vi "data_generation.vi"(0 "X Size":i32=8, 1 "slope":i16=10, 3 "scan range (um)":dbl=5.0, 4 "AmplitudeX":dbl=1.0, 5 "AmplitudeY":dbl=1.0, 6 "dwell time":i16=10, 7 "come back":i32, 8 "calibration":dbl=5.0, 9 "multicolor":dbl=5.0, 10 "zero point":dbl, 12 "first":dbl=0.5, 13 "Y size":i32=8, 15 "AmplitudeC":dbl=1.0, 17 "step size (um)":dbl=0.05, 18 "Samples per spot":i32=4, 19 "zero point 2":dbl) -> (2 "Output Graph":waveform(dbl)[](graph), 11 "DO":dbl[](array[numeric])=[0.0, 0.0, 0.0, 0.0, 0.0, 0.0, 0.0, 0.0, 1.0, 1.0, 1.0, 1.0, 1.0, 1.0, 1.0, 1.0, 2.0, 2.0, 2.0, 2.0, 2.0, 2.0, 2.0, 2.0, 3.0, 3.0, 3.0, 3.0, 3.0, 3.0, 3.0, 3.0, 4.0, 4.0, 4.0, 4.0, 4.0, 4.0, 4.0, 4.0, 5.0, 5.0, 5.0, 5.0, 5.0, 5.0, 5.0, 5.0, 6.0, 6.0, 6.0, 6.0, 6.0, 6.0, 6.0, 6.0, 7.0, 7.0, 7.0, 7.0, 7.0, 7.0, 7.0, 7.0, 7.0, 7.0, 7.0, 7.0, 7.0, 7.0, 7.0, 7.0, 6.0, 6.0, 6.0, 6.0, 6.0, 6.0, 6.0, 6.0, 5.0, 5.0, 5.0, 5.0, 5.0, 5.0, 5.0, 5.0, 4.0, 4.0, 4.0, 4.0, 4.0, 4.0, 4.0, 4.0, 3.0, 3.0, 3.0, 3.0, 3.0, 3.0, 3.0, 3.0, 2.0, 2.0, 2.0, 2.0, 2.0, 2.0, 2.0, 2.0, 1.0, 1.0, 1.0, 1.0, 1.0, 1.0, 1.0, 1.0, 0.0, 0.0, 0.0, 0.0, 0.0, 0.0, 0.0, 0.0], 14 "XY Scan":waveform(dbl)[](array[waveform])=[{"t0"=timestamp(3264022747.299 s since 1904-01-01), "dt"=0.015625, "Y"=[-1.0, -0.7142857142857143, -0.4285714285714286, -0.1428571428571429, 0.1428571428571428, 0.4285714285714286, 0.7142857142857142, 1.0, 1.0, 0.7142857142857142, 0.4285714285714286, 0.1428571428571428, -0.1428571428571429, -0.4285714285714286, -0.7142857142857143, -1.0, -1.0, -0.7142857142857143, -0.4285714285714286, -0.1428571428571429, 0.1428571428571428, 0.4285714285714286, 0.7142857142857142, 1.0, 1.0, 0.7142857142857142, 0.4285714285714286, 0.1428571428571428, -0.1428571428571429, -0.4285714285714286, -0.7142857142857143, -1.0, -1.0, -0.7142857142857143, -0.4285714285714286, -0.1428571428571429, 0.1428571428571428, 0.4285714285714286, 0.7142857142857142, 1.0, 1.0, 0.7142857142857142, 0.4285714285714286, 0.1428571428571428, -0.1428571428571429, -0.4285714285714286, -0.7142857142857143, -1.0, -1.0, -0.7142857142857143, -0.4285714285714286, -0.1428571428571429, 0.1428571428571428, 0.4285714285714286, 0.7142857142857142, 1.0, 1.0, 0.7142857142857142, 0.4285714285714286, 0.1428571428571428, -0.1428571428571429, -0.4285714285714286, -0.7142857142857143, -1.0, -1.0, -0.7142857142857143, -0.4285714285714286, -0.1428571428571429, 0.1428571428571428, 0.4285714285714286, 0.7142857142857142, 1.0, 1.0, 0.7142857142857142, 0.4285714285714286, 0.1428571428571428, -0.1428571428571429, -0.4285714285714286, -0.7142857142857143, -1.0, -1.0, -0.7142857142857143, -0.4285714285714286, -0.1428571428571429, 0.1428571428571428, 0.4285714285714286, 0.7142857142857142, 1.0, 1.0, 0.7142857142857142, 0.4285714285714286, 0.1428571428571428, -0.1428571428571429, -0.4285714285714286, -0.7142857142857143, -1.0, -1.0, -0.7142857142857143, -0.4285714285714286, -0.1428571428571429, 0.1428571428571428, 0.4285714285714286, 0.7142857142857142, 1.0, 1.0, 0.7142857142857142, 0.4285714285714286, 0.1428571428571428, -0.1428571428571429, -0.4285714285714286, -0.7142857142857143, -1.0, -1.0, -0.7142857142857143, -0.4285714285714286, -0.1428571428571429, 0.1428571428571428, 0.4285714285714286, 0.7142857142857142, 1.0, 1.0, 0.7142857142857142, 0.4285714285714286, 0.1428571428571428, -0.1428571428571429, -0.4285714285714286, -0.7142857142857143, -1.0]}, {"t0"=timestamp(3264022747.299 s since 1904-01-01), "dt"=0.015625, "Y"=[-1.0, -1.0, -1.0, -1.0, -1.0, -1.0, -1.0, -1.0, -0.7142857142857143, -0.7142857142857143, -0.7142857142857143, -0.7142857142857143, -0.7142857142857143, -0.7142857142857143, -0.7142857142857143, -0.7142857142857143, -0.4285714285714286, -0.4285714285714286, -0.4285714285714286, -0.4285714285714286, -0.4285714285714286, -0.4285714285714286, -0.4285714285714286, -0.4285714285714286, -0.1428571428571429, -0.1428571428571429, -0.1428571428571429, -0.1428571428571429, -0.1428571428571429, -0.1428571428571429, -0.1428571428571429, -0.1428571428571429, 0.1428571428571428, 0.1428571428571428, 0.1428571428571428, 0.1428571428571428, 0.1428571428571428, 0.1428571428571428, 0.1428571428571428, 0.1428571428571428, 0.4285714285714286, 0.4285714285714286, 0.4285714285714286, 0.4285714285714286, 0.4285714285714286, 0.4285714285714286, 0.4285714285714286, 0.4285714285714286, 0.7142857142857142, 0.7142857142857142, 0.7142857142857142, 0.7142857142857142, 0.7142857142857142, 0.7142857142857142, 0.7142857142857142, 0.7142857142857142, 1.0, 1.0, 1.0, 1.0, 1.0, 1.0, 1.0, 1.0, 1.0, 1.0, 1.0, 1.0, 1.0, 1.0, 1.0, 1.0, 0.7142857142857142, 0.7142857142857142, 0.7142857142857142, 0.7142857142857142, 0.7142857142857142, 0.7142857142857142, 0.7142857142857142, 0.7142857142857142, 0.4285714285714286, 0.4285714285714286, 0.4285714285714286, 0.4285714285714286, 0.4285714285714286, 0.4285714285714286, 0.4285714285714286, 0.4285714285714286, 0.1428571428571428, 0.1428571428571428, 0.1428571428571428, 0.1428571428571428, 0.1428571428571428, 0.1428571428571428, 0.1428571428571428, 0.1428571428571428, -0.1428571428571429, -0.1428571428571429, -0.1428571428571429, -0.1428571428571429, -0.1428571428571429, -0.1428571428571429, -0.1428571428571429, -0.1428571428571429, -0.4285714285714286, -0.4285714285714286, -0.4285714285714286, -0.4285714285714286, -0.4285714285714286, -0.4285714285714286, -0.4285714285714286, -0.4285714285714286, -0.7142857142857143, -0.7142857142857143, -0.7142857142857143, -0.7142857142857143, -0.7142857142857143, -0.7142857142857143, -0.7142857142857143, -0.7142857142857143, -1.0, -1.0, -1.0, -1.0, -1.0, -1.0, -1.0, -1.0]}])   [LabVIEW 2017]
uses:
  <vilib>/Analysis/3filter.llb/Zero Phase Filter (DBL).vi
  <vilib>/Analysis/NI_AALBase.lvlib
panel:
  out "AO Data":dbl[][](array[numeric])
  out "nanoZ output":dbl[](array[numeric])=[-1.0, -1.0, -1.0, -1.0, -1.0, -1.0, -1.0, -1.0, -0.7142857142857143, -0.7142857142857143, -0.7142857142857143, -0.7142857142857143, -0.7142857142857143, -0.7142857142857143, -0.7142857142857143, -0.7142857142857143, -0.4285714285714286, -0.4285714285714286, -0.4285714285714286, -0.4285714285714286, -0.4285714285714286, -0.4285714285714286, -0.4285714285714286, -0.4285714285714286, -0.1428571428571429, -0.1428571428571429, -0.1428571428571429, -0.1428571428571429, -0.1428571428571429, -0.1428571428571429, -0.1428571428571429, -0.1428571428571429, 0.1428571428571428, 0.1428571428571428, 0.1428571428571428, 0.1428571428571428, 0.1428571428571428, 0.1428571428571428, 0.1428571428571428, 0.1428571428571428, 0.4285714285714286, 0.4285714285714286, 0.4285714285714286, 0.4285714285714286, 0.4285714285714286, 0.4285714285714286, 0.4285714285714286, 0.4285714285714286, 0.7142857142857142, 0.7142857142857142, 0.7142857142857142, 0.7142857142857142, 0.7142857142857142, 0.7142857142857142, 0.7142857142857142, 0.7142857142857142, 1.0, 1.0, 1.0, 1.0, 1.0, 1.0, 1.0, 1.0, 1.0, 1.0, 1.0, 1.0, 1.0, 1.0, 1.0, 1.0, 0.7142857142857142, 0.7142857142857142, 0.7142857142857142, 0.7142857142857142, 0.7142857142857142, 0.7142857142857142, 0.7142857142857142, 0.7142857142857142, 0.4285714285714286, 0.4285714285714286, 0.4285714285714286, 0.4285714285714286, 0.4285714285714286, 0.4285714285714286, 0.4285714285714286, 0.4285714285714286, 0.1428571428571428, 0.1428571428571428, 0.1428571428571428, 0.1428571428571428, 0.1428571428571428, 0.1428571428571428, 0.1428571428571428, 0.1428571428571428, -0.1428571428571429, -0.1428571428571429, -0.1428571428571429, -0.1428571428571429, -0.1428571428571429, -0.1428571428571429, -0.1428571428571429, -0.1428571428571429, -0.4285714285714286, -0.4285714285714286, -0.4285714285714286, -0.4285714285714286, -0.4285714285714286, -0.4285714285714286, -0.4285714285714286, -0.4285714285714286, -0.7142857142857143, -0.7142857142857143, -0.7142857142857143, -0.7142857142857143, -0.7142857142857143, -0.7142857142857143, -0.7142857142857143, -0.7142857142857143, -1.0, -1.0, -1.0, -1.0, -1.0, -1.0, -1.0, -1.0]
  out "nanoZ":dbl[](array[numeric])=[0.0, 1.0, 2.0, 3.0, 4.0, 5.0, 6.0, 7.0, 7.0, 6.0, 5.0, 4.0, 3.0, 2.0, 1.0, 0.0, 0.0, 1.0, 2.0, 3.0, 4.0, 5.0, 6.0, 7.0, 7.0, 6.0, 5.0, 4.0, 3.0, 2.0, 1.0, 0.0, 0.0, 1.0, 2.0, 3.0, 4.0, 5.0, 6.0, 7.0, 7.0, 6.0, 5.0, 4.0, 3.0, 2.0, 1.0, 0.0, 0.0, 1.0, 2.0, 3.0, 4.0, 5.0, 6.0, 7.0, 7.0, 6.0, 5.0, 4.0, 3.0, 2.0, 1.0, 0.0, 0.0, 1.0, 2.0, 3.0, 4.0, 5.0, 6.0, 7.0, 7.0, 6.0, 5.0, 4.0, 3.0, 2.0, 1.0, 0.0, 0.0, 1.0, 2.0, 3.0, 4.0, 5.0, 6.0, 7.0, 7.0, 6.0, 5.0, 4.0, 3.0, 2.0, 1.0, 0.0, 0.0, 1.0, 2.0, 3.0, 4.0, 5.0, 6.0, 7.0, 7.0, 6.0, 5.0, 4.0, 3.0, 2.0, 1.0, 0.0, 0.0, 1.0, 2.0, 3.0, 4.0, 5.0, 6.0, 7.0, 7.0, 6.0, 5.0, 4.0, 3.0, 2.0, 1.0, 0.0]
  out "Trigger output":dbl[](array[numeric])=[-1.0, -1.0, -1.0, -1.0, -1.0, -1.0, -1.0, -1.0, -0.7142857142857143, -0.7142857142857143, -0.7142857142857143, -0.7142857142857143, -0.7142857142857143, -0.7142857142857143, -0.7142857142857143, -0.7142857142857143, -0.4285714285714286, -0.4285714285714286, -0.4285714285714286, -0.4285714285714286, -0.4285714285714286, -0.4285714285714286, -0.4285714285714286, -0.4285714285714286, -0.1428571428571429, -0.1428571428571429, -0.1428571428571429, -0.1428571428571429, -0.1428571428571429, -0.1428571428571429, -0.1428571428571429, -0.1428571428571429, 0.1428571428571428, 0.1428571428571428, 0.1428571428571428, 0.1428571428571428, 0.1428571428571428, 0.1428571428571428, 0.1428571428571428, 0.1428571428571428, 0.4285714285714286, 0.4285714285714286, 0.4285714285714286, 0.4285714285714286, 0.4285714285714286, 0.4285714285714286, 0.4285714285714286, 0.4285714285714286, 0.7142857142857142, 0.7142857142857142, 0.7142857142857142, 0.7142857142857142, 0.7142857142857142, 0.7142857142857142, 0.7142857142857142, 0.7142857142857142, 1.0, 1.0, 1.0, 1.0, 1.0, 1.0, 1.0, 1.0, 1.0, 1.0, 1.0, 1.0, 1.0, 1.0, 1.0, 1.0, 0.7142857142857142, 0.7142857142857142, 0.7142857142857142, 0.7142857142857142, 0.7142857142857142, 0.7142857142857142, 0.7142857142857142, 0.7142857142857142, 0.4285714285714286, 0.4285714285714286, 0.4285714285714286, 0.4285714285714286, 0.4285714285714286, 0.4285714285714286, 0.4285714285714286, 0.4285714285714286, 0.1428571428571428, 0.1428571428571428, 0.1428571428571428, 0.1428571428571428, 0.1428571428571428, 0.1428571428571428, 0.1428571428571428, 0.1428571428571428, -0.1428571428571429, -0.1428571428571429, -0.1428571428571429, -0.1428571428571429, -0.1428571428571429, -0.1428571428571429, -0.1428571428571429, -0.1428571428571429, -0.4285714285714286, -0.4285714285714286, -0.4285714285714286, -0.4285714285714286, -0.4285714285714286, -0.4285714285714286, -0.4285714285714286, -0.4285714285714286, -0.7142857142857143, -0.7142857142857143, -0.7142857142857143, -0.7142857142857143, -0.7142857142857143, -0.7142857142857143, -0.7142857142857143, -0.7142857142857143, -1.0, -1.0, -1.0, -1.0, -1.0, -1.0, -1.0, -1.0]
  out "Trigger":dbl[](array[numeric])=[0.0, 0.0, 0.0, 0.0, 0.0, 0.0, 0.0, 0.0, 1.0, 1.0, 1.0, 1.0, 1.0, 1.0, 1.0, 1.0, 2.0, 2.0, 2.0, 2.0, 2.0, 2.0, 2.0, 2.0, 3.0, 3.0, 3.0, 3.0, 3.0, 3.0, 3.0, 3.0, 4.0, 4.0, 4.0, 4.0, 4.0, 4.0, 4.0, 4.0, 5.0, 5.0, 5.0, 5.0, 5.0, 5.0, 5.0, 5.0, 6.0, 6.0, 6.0, 6.0, 6.0, 6.0, 6.0, 6.0, 7.0, 7.0, 7.0, 7.0, 7.0, 7.0, 7.0, 7.0, 7.0, 7.0, 7.0, 7.0, 7.0, 7.0, 7.0, 7.0, 6.0, 6.0, 6.0, 6.0, 6.0, 6.0, 6.0, 6.0, 5.0, 5.0, 5.0, 5.0, 5.0, 5.0, 5.0, 5.0, 4.0, 4.0, 4.0, 4.0, 4.0, 4.0, 4.0, 4.0, 3.0, 3.0, 3.0, 3.0, 3.0, 3.0, 3.0, 3.0, 2.0, 2.0, 2.0, 2.0, 2.0, 2.0, 2.0, 2.0, 1.0, 1.0, 1.0, 1.0, 1.0, 1.0, 1.0, 1.0, 0.0, 0.0, 0.0, 0.0, 0.0, 0.0, 0.0, 0.0]
  in  "dt":dbl=1e-05
  out "time":dbl=3264022747.299 format="%<%I:%M:%S %p\n%m/%d/%Y>T"
  out "Y output Array":dbl[](array[numeric])=[-1.0, -1.0, -1.0, -1.0, -1.0, -1.0, -1.0, -1.0, -0.7142857142857143, -0.7142857142857143, -0.7142857142857143, -0.7142857142857143, -0.7142857142857143, -0.7142857142857143, -0.7142857142857143, -0.7142857142857143, -0.4285714285714286, -0.4285714285714286, -0.4285714285714286, -0.4285714285714286, -0.4285714285714286, -0.4285714285714286, -0.4285714285714286, -0.4285714285714286, -0.1428571428571429, -0.1428571428571429, -0.1428571428571429, -0.1428571428571429, -0.1428571428571429, -0.1428571428571429, -0.1428571428571429, -0.1428571428571429, 0.1428571428571428, 0.1428571428571428, 0.1428571428571428, 0.1428571428571428, 0.1428571428571428, 0.1428571428571428, 0.1428571428571428, 0.1428571428571428, 0.4285714285714286, 0.4285714285714286, 0.4285714285714286, 0.4285714285714286, 0.4285714285714286, 0.4285714285714286, 0.4285714285714286, 0.4285714285714286, 0.7142857142857142, 0.7142857142857142, 0.7142857142857142, 0.7142857142857142, 0.7142857142857142, 0.7142857142857142, 0.7142857142857142, 0.7142857142857142, 1.0, 1.0, 1.0, 1.0, 1.0, 1.0, 1.0, 1.0, 1.0, 1.0, 1.0, 1.0, 1.0, 1.0, 1.0, 1.0, 0.7142857142857142, 0.7142857142857142, 0.7142857142857142, 0.7142857142857142, 0.7142857142857142, 0.7142857142857142, 0.7142857142857142, 0.7142857142857142, 0.4285714285714286, 0.4285714285714286, 0.4285714285714286, 0.4285714285714286, 0.4285714285714286, 0.4285714285714286, 0.4285714285714286, 0.4285714285714286, 0.1428571428571428, 0.1428571428571428, 0.1428571428571428, 0.1428571428571428, 0.1428571428571428, 0.1428571428571428, 0.1428571428571428, 0.1428571428571428, -0.1428571428571429, -0.1428571428571429, -0.1428571428571429, -0.1428571428571429, -0.1428571428571429, -0.1428571428571429, -0.1428571428571429, -0.1428571428571429, -0.4285714285714286, -0.4285714285714286, -0.4285714285714286, -0.4285714285714286, -0.4285714285714286, -0.4285714285714286, -0.4285714285714286, -0.4285714285714286, -0.7142857142857143, -0.7142857142857143, -0.7142857142857143, -0.7142857142857143, -0.7142857142857143, -0.7142857142857143, -0.7142857142857143, -0.7142857142857143, -1.0, -1.0, -1.0, -1.0, -1.0, -1.0, -1.0, -1.0]
  out "X output Array":dbl[](array[numeric])=[-1.0, -0.7142857142857143, -0.4285714285714286, -0.1428571428571429, 0.1428571428571428, 0.4285714285714286, 0.7142857142857142, 1.0, 1.0, 0.7142857142857142, 0.4285714285714286, 0.1428571428571428, -0.1428571428571429, -0.4285714285714286, -0.7142857142857143, -1.0, -1.0, -0.7142857142857143, -0.4285714285714286, -0.1428571428571429, 0.1428571428571428, 0.4285714285714286, 0.7142857142857142, 1.0, 1.0, 0.7142857142857142, 0.4285714285714286, 0.1428571428571428, -0.1428571428571429, -0.4285714285714286, -0.7142857142857143, -1.0, -1.0, -0.7142857142857143, -0.4285714285714286, -0.1428571428571429, 0.1428571428571428, 0.4285714285714286, 0.7142857142857142, 1.0, 1.0, 0.7142857142857142, 0.4285714285714286, 0.1428571428571428, -0.1428571428571429, -0.4285714285714286, -0.7142857142857143, -1.0, -1.0, -0.7142857142857143, -0.4285714285714286, -0.1428571428571429, 0.1428571428571428, 0.4285714285714286, 0.7142857142857142, 1.0, 1.0, 0.7142857142857142, 0.4285714285714286, 0.1428571428571428, -0.1428571428571429, -0.4285714285714286, -0.7142857142857143, -1.0, -1.0, -0.7142857142857143, -0.4285714285714286, -0.1428571428571429, 0.1428571428571428, 0.4285714285714286, 0.7142857142857142, 1.0, 1.0, 0.7142857142857142, 0.4285714285714286, 0.1428571428571428, -0.1428571428571429, -0.4285714285714286, -0.7142857142857143, -1.0, -1.0, -0.7142857142857143, -0.4285714285714286, -0.1428571428571429, 0.1428571428571428, 0.4285714285714286, 0.7142857142857142, 1.0, 1.0, 0.7142857142857142, 0.4285714285714286, 0.1428571428571428, -0.1428571428571429, -0.4285714285714286, -0.7142857142857143, -1.0, -1.0, -0.7142857142857143, -0.4285714285714286, -0.1428571428571429, 0.1428571428571428, 0.4285714285714286, 0.7142857142857142, 1.0, 1.0, 0.7142857142857142, 0.4285714285714286, 0.1428571428571428, -0.1428571428571429, -0.4285714285714286, -0.7142857142857143, -1.0, -1.0, -0.7142857142857143, -0.4285714285714286, -0.1428571428571429, 0.1428571428571428, 0.4285714285714286, 0.7142857142857142, 1.0, 1.0, 0.7142857142857142, 0.4285714285714286, 0.1428571428571428, -0.1428571428571429, -0.4285714285714286, -0.7142857142857143, -1.0]
  out "Y index Array":dbl[](array[numeric])=[0.0, 0.0, 0.0, 0.0, 0.0, 0.0, 0.0, 0.0, 1.0, 1.0, 1.0, 1.0, 1.0, 1.0, 1.0, 1.0, 2.0, 2.0, 2.0, 2.0, 2.0, 2.0, 2.0, 2.0, 3.0, 3.0, 3.0, 3.0, 3.0, 3.0, 3.0, 3.0, 4.0, 4.0, 4.0, 4.0, 4.0, 4.0, 4.0, 4.0, 5.0, 5.0, 5.0, 5.0, 5.0, 5.0, 5.0, 5.0, 6.0, 6.0, 6.0, 6.0, 6.0, 6.0, 6.0, 6.0, 7.0, 7.0, 7.0, 7.0, 7.0, 7.0, 7.0, 7.0, 7.0, 7.0, 7.0, 7.0, 7.0, 7.0, 7.0, 7.0, 6.0, 6.0, 6.0, 6.0, 6.0, 6.0, 6.0, 6.0, 5.0, 5.0, 5.0, 5.0, 5.0, 5.0, 5.0, 5.0, 4.0, 4.0, 4.0, 4.0, 4.0, 4.0, 4.0, 4.0, 3.0, 3.0, 3.0, 3.0, 3.0, 3.0, 3.0, 3.0, 2.0, 2.0, 2.0, 2.0, 2.0, 2.0, 2.0, 2.0, 1.0, 1.0, 1.0, 1.0, 1.0, 1.0, 1.0, 1.0, 0.0, 0.0, 0.0, 0.0, 0.0, 0.0, 0.0, 0.0]
  out "X index Array":dbl[](array[numeric])=[0.0, 1.0, 2.0, 3.0, 4.0, 5.0, 6.0, 7.0, 7.0, 6.0, 5.0, 4.0, 3.0, 2.0, 1.0, 0.0, 0.0, 1.0, 2.0, 3.0, 4.0, 5.0, 6.0, 7.0, 7.0, 6.0, 5.0, 4.0, 3.0, 2.0, 1.0, 0.0, 0.0, 1.0, 2.0, 3.0, 4.0, 5.0, 6.0, 7.0, 7.0, 6.0, 5.0, 4.0, 3.0, 2.0, 1.0, 0.0, 0.0, 1.0, 2.0, 3.0, 4.0, 5.0, 6.0, 7.0, 7.0, 6.0, 5.0, 4.0, 3.0, 2.0, 1.0, 0.0, 0.0, 1.0, 2.0, 3.0, 4.0, 5.0, 6.0, 7.0, 7.0, 6.0, 5.0, 4.0, 3.0, 2.0, 1.0, 0.0, 0.0, 1.0, 2.0, 3.0, 4.0, 5.0, 6.0, 7.0, 7.0, 6.0, 5.0, 4.0, 3.0, 2.0, 1.0, 0.0, 0.0, 1.0, 2.0, 3.0, 4.0, 5.0, 6.0, 7.0, 7.0, 6.0, 5.0, 4.0, 3.0, 2.0, 1.0, 0.0, 0.0, 1.0, 2.0, 3.0, 4.0, 5.0, 6.0, 7.0, 7.0, 6.0, 5.0, 4.0, 3.0, 2.0, 1.0, 0.0]
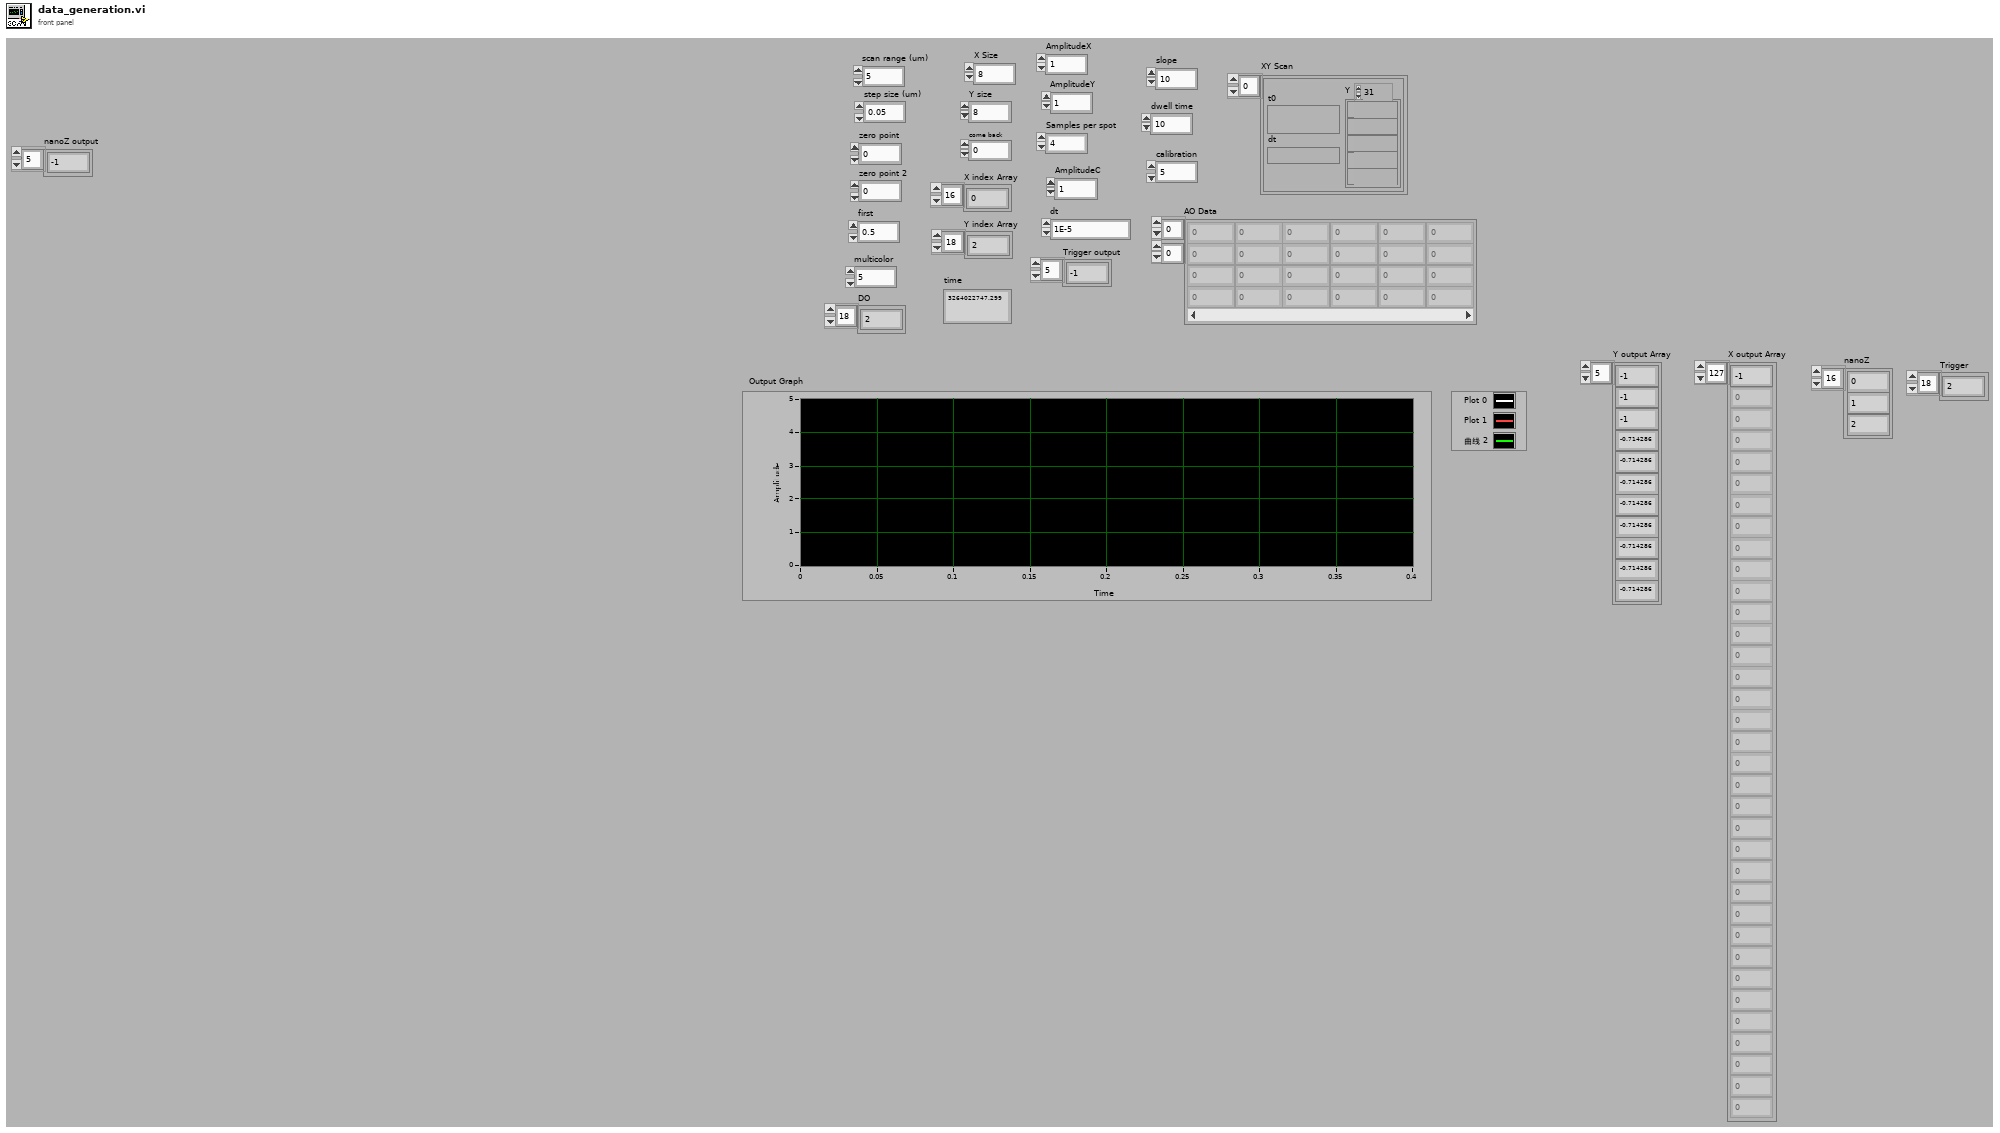
[diagram p1: front panel]
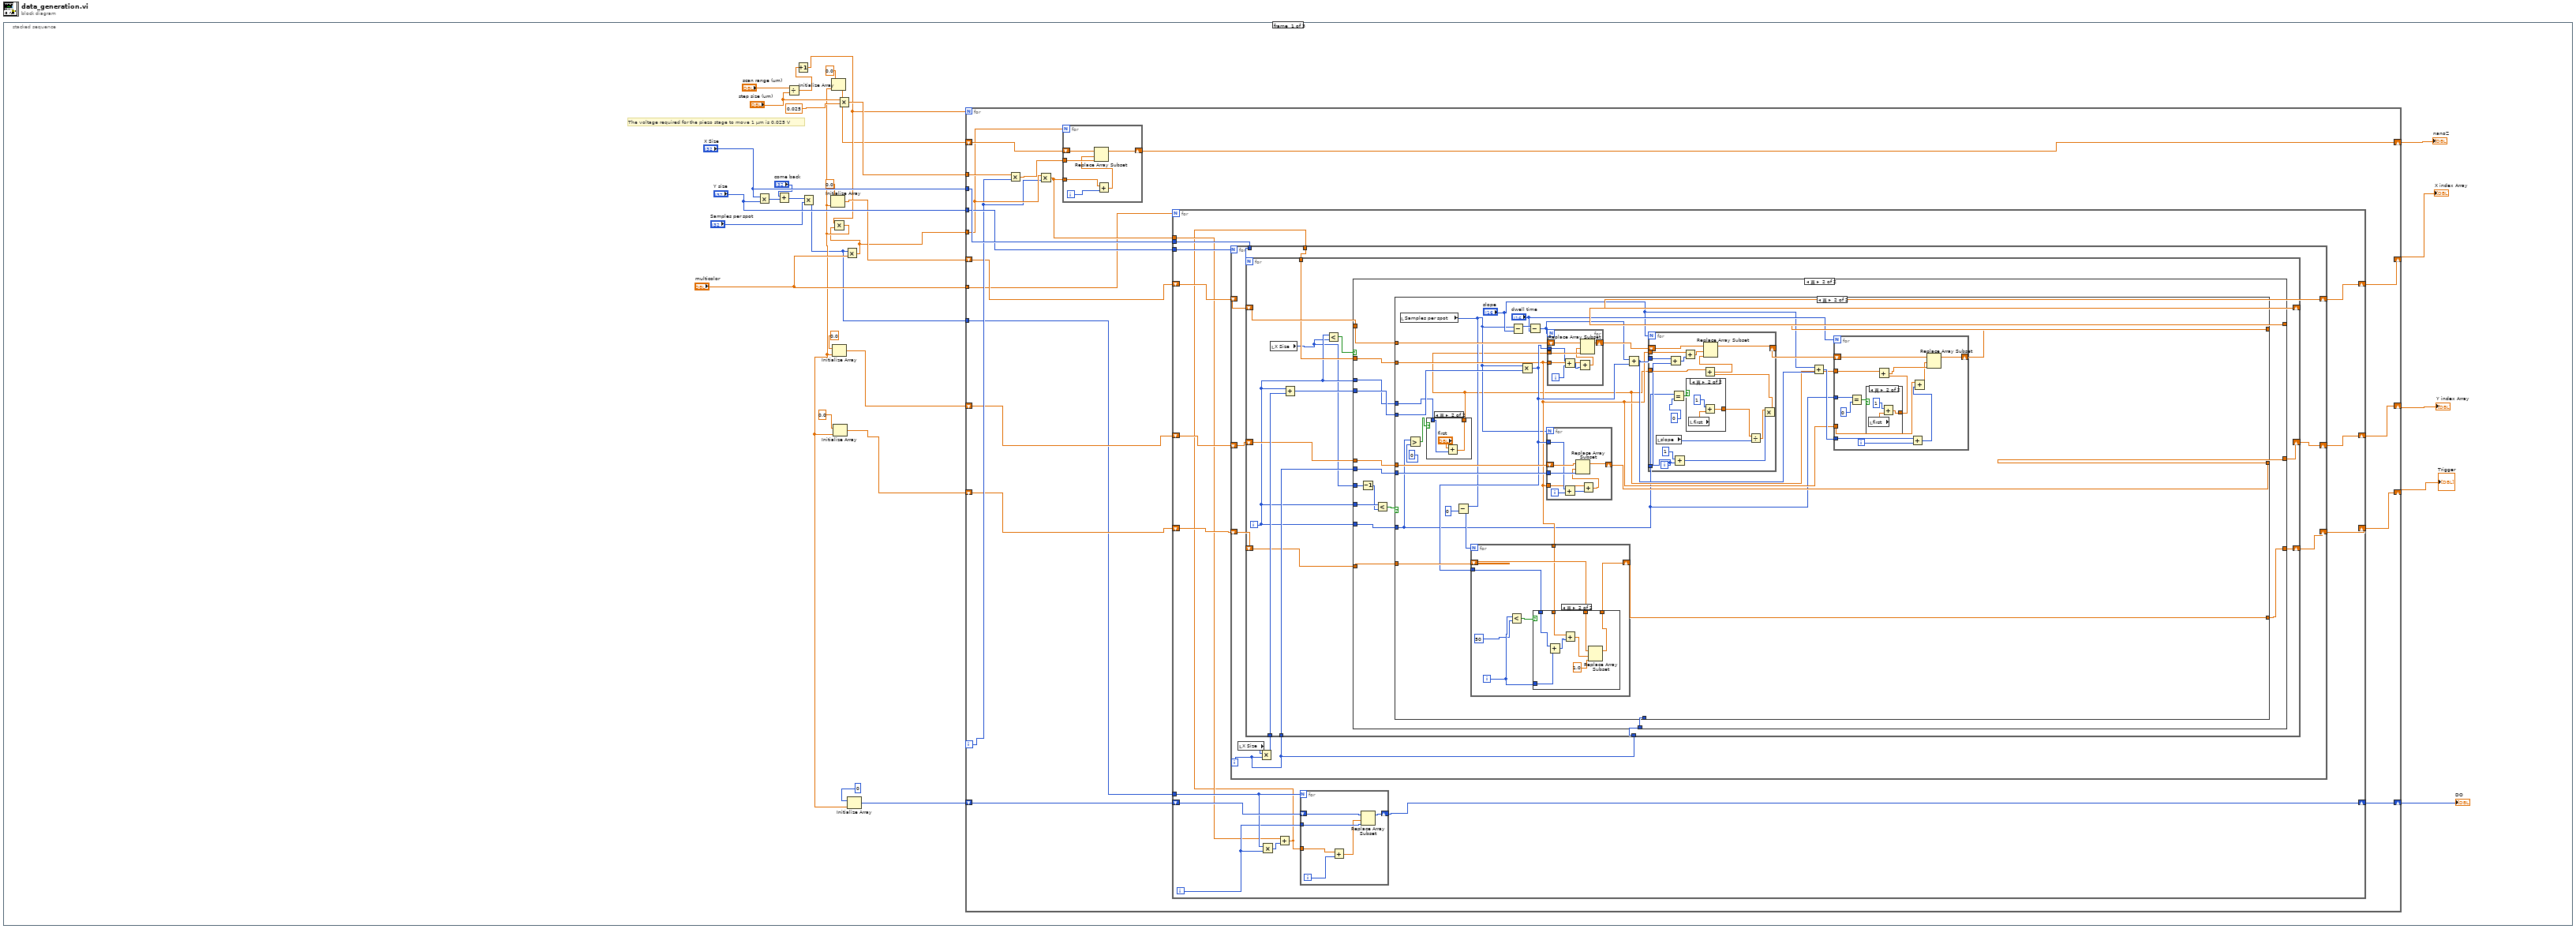
[diagram p0: block diagram]
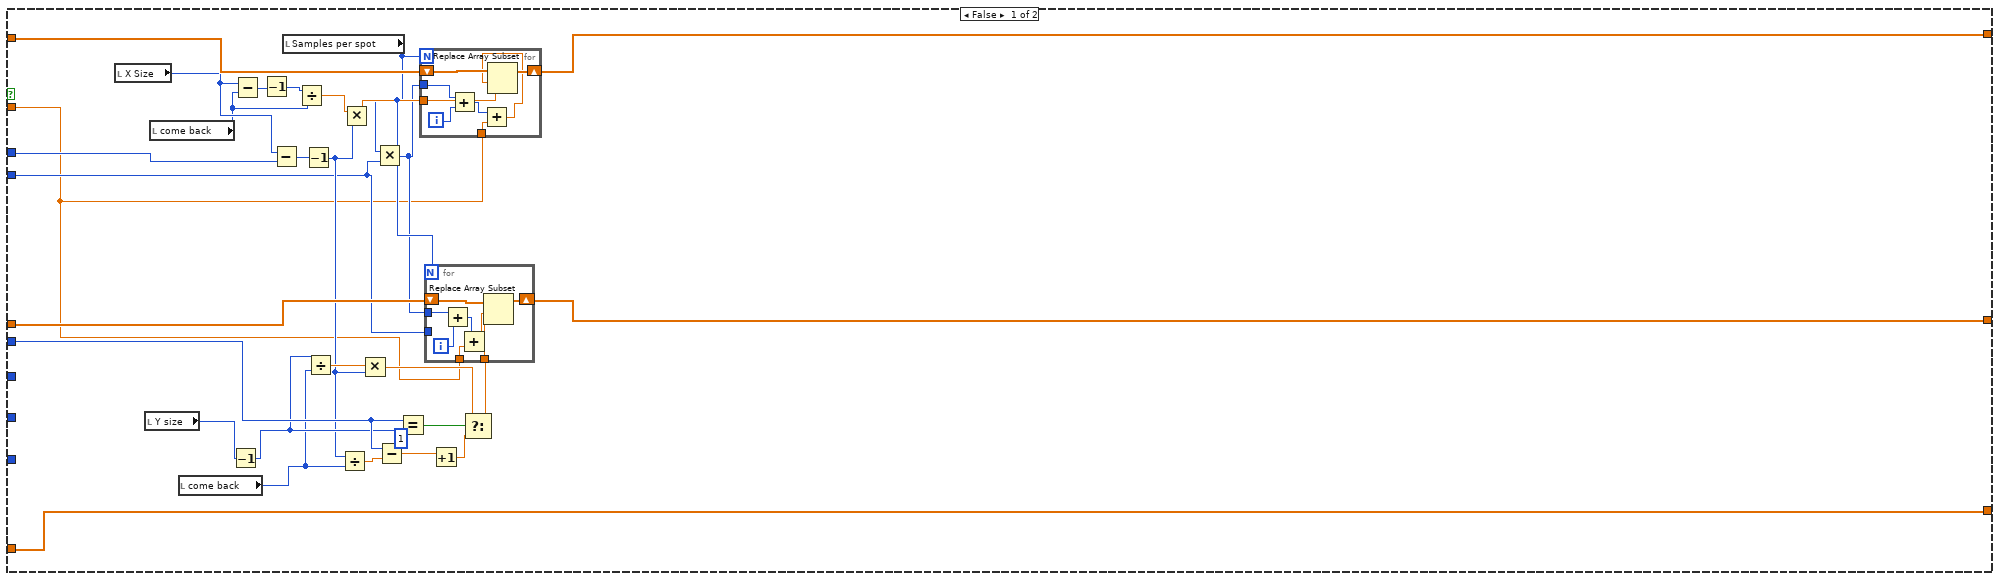
[diagram p2: hidden frame]
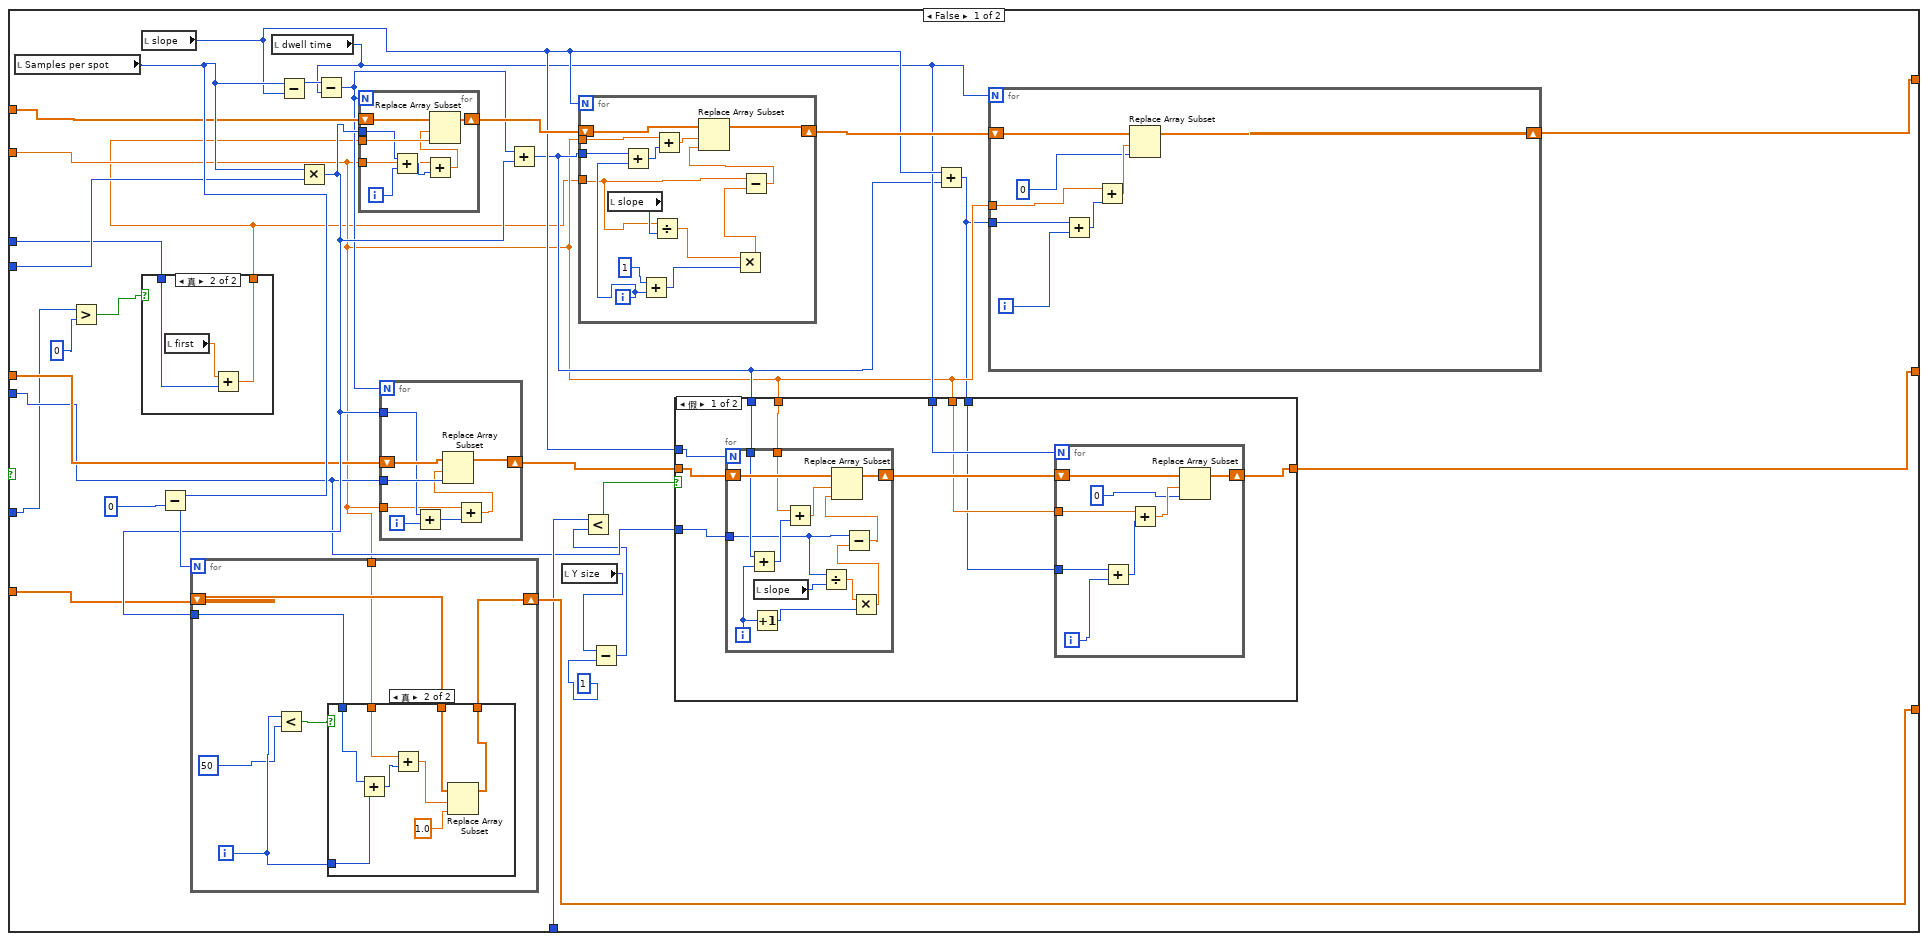
[diagram p3: hidden frame]
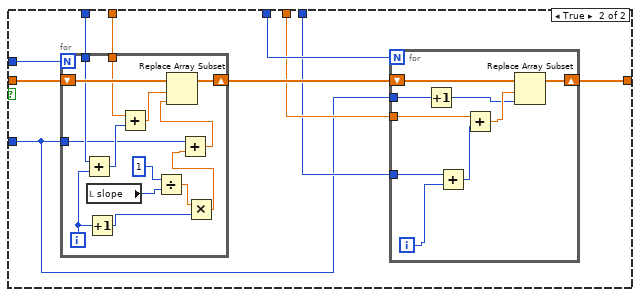
[diagram p5: hidden frame]
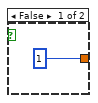
[diagram p8: hidden frame]
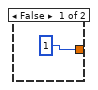
[diagram p9: hidden frame]
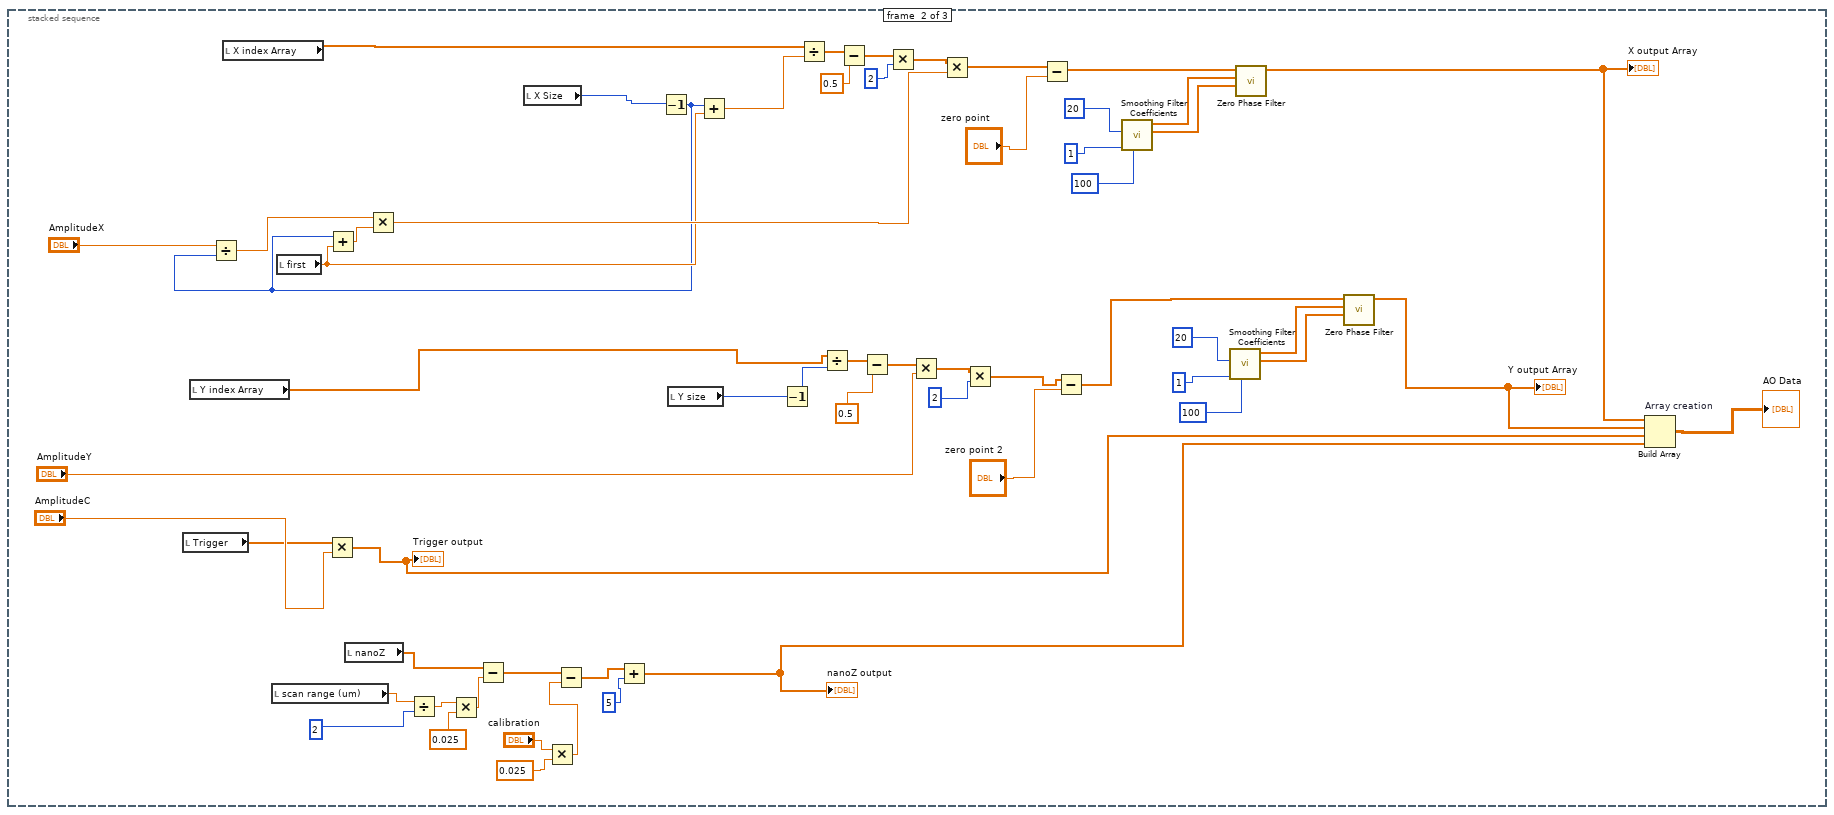
[diagram p11: hidden frame]
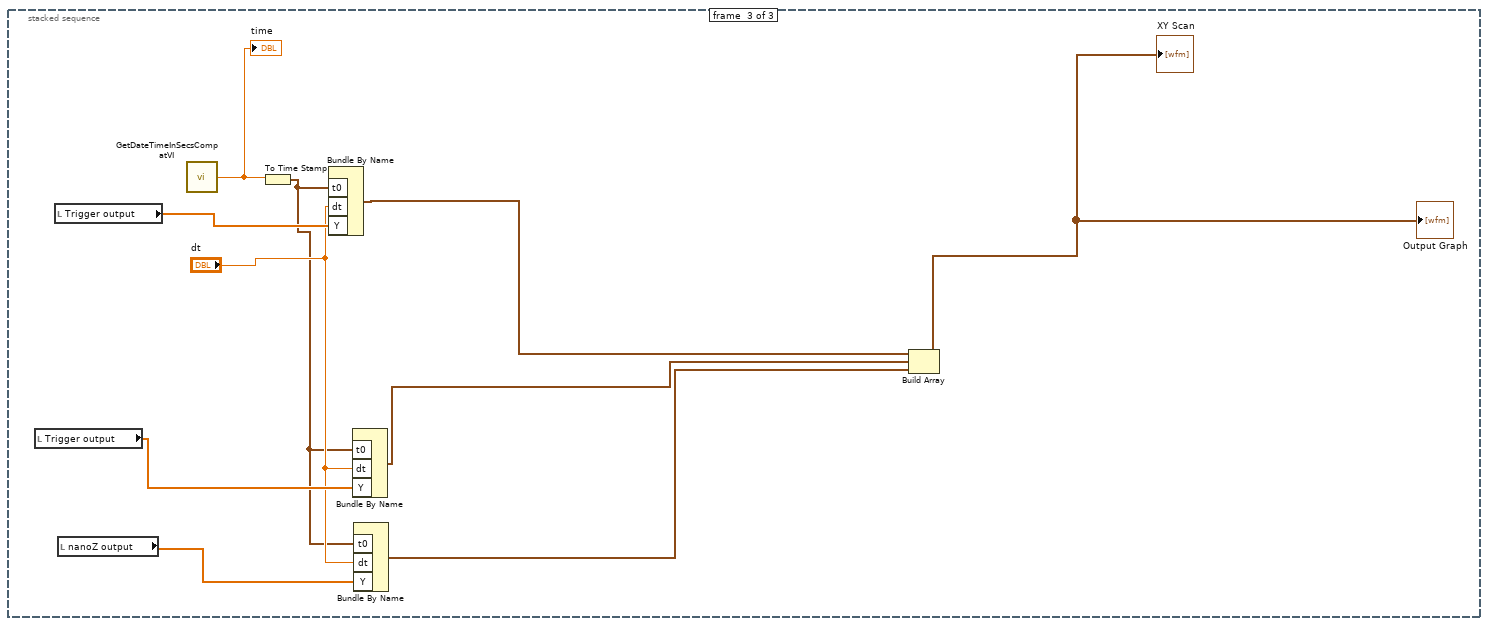
[diagram p12: hidden frame]
diagram:
  n1 = stacked-sequence {
    frame #0 {
      # "The voltage required for the piezo stage to move 1 μm is 0.025 V"
      n2 = Multiply(x="X Size", y="Y size") -> (x*y=w9:i32)
      n3 = Add(x="come back", y=w9) -> (x+y=w8:i32)
      n4 = Divide(x="scan range (um)", y="step size (um)") -> (x/y=w16:dbl)
      n5 = Increment(x=w16) -> (x+1=w17:dbl)
      n6 = Multiply(x=w8, y="Samples per spot") -> (x*y=w1:i32)
      n7 = Multiply(x="step size (um)", y=0.025) -> (x*y=w19:dbl)
      n8 = Multiply(x=w1, y="multicolor") -> (x*y=w2:dbl)
      n9 = Multiply(x=w17, y=w2) -> (x*y=w3:dbl)
      n10 = Initialize Array(0.0, w3) -> (w22:dbl[])
      n11 = Initialize Array(0.0, w3) -> (w11:dbl[])
      n12 = Initialize Array(0.0, w3) -> (w23:dbl[])
      n13 = Initialize Array(0.0, w3) -> (w24:dbl[])
      n14 = Initialize Array(0, w3) -> (w6:i32[])
      n15 = for {
        N: w17 -> [_]
        tunnel: "X Size" -> [w48]
        tunnel: "Y size" -> [w47]
        shift-right: [w50] -> w13
        shift-left: w23 -> [w38]
        shift-right: [w37] -> w12
        shift-left: w24 -> [w36]
        shift-right: [w49] -> w14
        shift-left: w22 -> [w39]
        tunnel: w19 -> [w46]
        tunnel: w2 -> [w42]
        shift-right: [w43] -> w15
        shift-left: w11 -> [w45]
        tunnel: "multicolor" -> [w35]
        shift-right: [w33] -> w5
        shift-left: w6 -> [w34]
        tunnel: w1 -> [w32]
        i -> [w41]
        n16 = Multiply(x=w46, y=w41) -> (x*y=w44:dbl)
        n17 = Multiply(x=w42, y=w41) -> (x*y=w40:dbl)
        n18 = for {
          N: w42 -> [_]
          shift-right: [w417] -> w43
          shift-left: w45 -> [w418]
          tunnel: w44 -> [w416]
          tunnel: w40 -> [w413]
          i -> [w415]
          n19 = Add(x=w413, y=w415) -> (x+y=w414:dbl)
          n20 = Replace Array Subset(array=w418, new element=w416, index=w414) -> (w417:dbl[])
        }
        n21 = for {
          N: w35 -> [_]
          tunnel: w48 -> [w63]
          tunnel: w47 -> [w62]
          tunnel: w40 -> [w52]
          shift-right: [w64] -> w49
          shift-left: w39 -> [w61]
          shift-right: [w65] -> w50
          shift-left: w38 -> [w60]
          shift-right: [w59] -> w37
          shift-left: w36 -> [w58]
          shift-right: [w56] -> w33
          shift-left: w34 -> [w57]
          tunnel: w32 -> [w55]
          i -> [w54]
          n22 = Multiply(x=w55, y=w54) -> (x*y=w53:i32)
          n23 = Add(x=w52, y=w53) -> (x+y=w51:dbl)
          n24 = for {
            N: w62 -> [_]
            tunnel: w63 -> [w82]
            shift-right: [w80] -> w64
            shift-left: w61 -> [w81]
            shift-right: [w76] -> w65
            shift-left: w60 -> [w77]
            shift-right: [w74] -> w59
            shift-left: w58 -> [w75]
            tunnel: w51 -> [w73]
            i -> [w72]
            n25 = local read "X Size"() -> (w79:i32)
            n26 = Multiply(x=w79, y=w72) -> (x*y=w78:i32)
            n27 = for {
              N: w82 -> [_]
              shift-right: [w95] -> w80
              shift-left: w81 -> [w96]
              tunnel: w78 -> [w94]
              shift-right: [w90] -> w76
              shift-left: w77 -> [w91]
              tunnel: w72 -> [w89]
              shift-right: [w83] -> w74
              shift-left: w75 -> [w88]
              tunnel: w73 -> [w87]
              tunnel: w72 -> [w86]
              i -> [w85]
              n28 = local read "X Size"() -> (w84:i32)
              n29 = Add(x=w85, y=w94) -> (x+y=w93:i32)
              n30 = Less?(x=w85, y=w84) -> (x < y?=w92:bool)
              n31 = case shown="真" w92 {
                tunnel: w96 -> [w125 w157]
                tunnel: [w124 w151] -> w95
                tunnel: w93 -> [w103 w153]
                tunnel: w85 -> [w119 w150]
                tunnel: w91 -> [w115 w156]
                tunnel: [w114 w155] -> w90
                tunnel: w89 -> [w111 w154]
                tunnel: w88 -> [w97 w152]
                tunnel: w85 -> [_ w149]
                tunnel: w84 -> [_ w147]
                tunnel: w87 -> [w98 w145]
                tunnel: w86 -> [_ w144]
                tunnel: w85 -> [_ w143]
                tunnel: [w97 w142] -> w83
                frame False {
                  (unwired) 1
                  n32 = local read "X Size"() -> (w118:i32)
                  n33 = local read "Y size"() -> (w99:i32)
                  n34 = local read "come back"() -> (w116:i32)
                  n35 = local read "come back"() -> (w100:i32)
                  n36 = Decrement(x=w99) -> (x-1=w107:i32)
                  n37 = Subtract(x=w118, y=w116) -> (x-y=w123:i32)
                  n38 = Decrement(x=w123) -> (x-1=w122:i32)
                  n39 = Subtract(x=w118, y=w119) -> (x-y=w120:i32)
                  n40 = local read "Samples per spot"() -> (w102:i32)
                  n41 = Divide(x=w122, y=w116) -> (x/y=w121:dbl)
                  n42 = Decrement(x=w120) -> (x-1=w105:i32)
                  n43 = Divide(x=w107, y=w100) -> (x/y=w106:dbl)
                  n44 = Divide(x=w105, y=w100) -> (x/y=w112:dbl)
                  n45 = Multiply(x=w121, y=w105) -> (x*y=w117:dbl)
                  n46 = Multiply(x=w106, y=w105) -> (x*y=w104:dbl)
                  n47 = Multiply(x=w102, y=w103) -> (x*y=w101:i32)
                  n48 = Subtract(x=w111, y=w112) -> (x-y=w109:dbl)
                  n49 = Equal?(x=w111, y=w107) -> (x = y?=w113:bool)
                  n50 = for {
                    N: w102 -> [_]
                    tunnel: w117 -> [w139]
                    shift-right: [w140] -> w124
                    shift-left: w125 -> [w141]
                    tunnel: w101 -> [w137]
                    tunnel: w98 -> [w134]
                    i -> [w138]
                    n51 = Add(x=w137, y=w138) -> (x+y=w136:i32)
                    n52 = Add(x=w136, y=w134) -> (x+y=w135:dbl)
                    n53 = Replace Array Subset(array=w141, new element=w139, index=w135) -> (w140:dbl[])
                  }
                  n54 = Increment(x=w109) -> (x+1=w108:dbl)
                  n55 = Select(t=w104, s=w113, f=w108) -> (s? t:f=w110:dbl)
                  n56 = for {
                    N: w102 -> [_]
                    tunnel: w103 -> [_]
                    tunnel: w110 -> [w131]
                    shift-right: [w132] -> w114
                    shift-left: w115 -> [w133]
                    tunnel: w101 -> [w130]
                    tunnel: w98 -> [w126]
                    i -> [w129]
                    n57 = Add(x=w130, y=w129) -> (x+y=w128:i32)
                    n58 = Add(x=w128, y=w126) -> (x+y=w127:dbl)
                    n59 = Replace Array Subset(array=w133, new element=w131, index=w127) -> (w132:dbl[])
                  }
                }
                frame True {
                  n60 = Decrement(x=w147) -> (x-1=w148:i32)
                  n61 = Less?(x=w149, y=w148) -> (x < y?=w146:bool)
                  n62 = case shown="真" w146 {
                    tunnel: w157 -> [w182 w337]
                    tunnel: w156 -> [w180 w336]
                    tunnel: [w161 w335] -> w155
                    tunnel: w154 -> [w171 w334]
                    tunnel: w153 -> [w181 w333]
                    tunnel: w152 -> [w179 w332]
                    tunnel: [w178 w329] -> w142
                    tunnel: [w162 w325] -> w151
                    tunnel: w150 -> [w167 w315]
                    tunnel: w145 -> [w170 w318]
                    tunnel: w144 -> [w177 _]
                    tunnel: w143 -> [w165 w314]
                    frame False {
                      n63 = local read "Samples per spot"() -> (w183:i32)
                      n64 = Greater?(x=w165, y=0) -> (0:w164:bool)
                      n65 = local read "slope"() -> (w174:i16)
                      n66 = case shown="真" w164 {
                        tunnel: [w190 w191] -> w168
                        tunnel: w167 -> [w190 w192]
                        frame False {
                        }
                        frame True {
                          n67 = local read "first"() -> (w193:dbl)
                          n68 = Add(x=w193, y=w192) -> (x+y=w191:dbl)
                        }
                      }
                      n69 = Subtract(x=w183, y=0) -> (x-y=w189:i32)
                      n70 = local read "dwell time"() -> (w173:i16)
                      n71 = Subtract(x=w183, y=w174) -> (x-y=w184:i32)
                      n72 = Multiply(x=w183, y=w181) -> (x*y=w186:i32)
                      n73 = for {
                        N: w189 -> [_]
                        tunnel: w186 -> [w286]
                        shift-right: [w285] -> w178
                        shift-left: w179 -> [w284]
                        tunnel: w170 -> [w280]
                        i -> [w283]
                        n74 = Less?(x=w283, y=50) -> (x < y?=w281:bool)
                        n75 = case shown="真" w281 {
                          tunnel: w286 -> [_ w294]
                          tunnel: [w287 w293] -> w285
                          tunnel: w283 -> [_ w292]
                          tunnel: w284 -> [w287 w291]
                          tunnel: w280 -> [_ w288]
                          frame False {
                          }
                          frame True {
                            n76 = Add(x=w294, y=w292) -> (x+y=w289:i32)
                            n77 = Add(x=w288, y=w289) -> (x+y=w290:dbl)
                            n78 = Replace Array Subset(array=w291, new element=1.0 ("新元素/子数组"), index=w290) -> (w293:dbl[])
                          }
                        }
                      }
                      n79 = Subtract(x=w184, y=w173) -> (x-y=w175:i32)
                      n80 = for {
                        N: w175 -> [_]
                        tunnel: w168 -> [w309]
                        tunnel: w186 -> [w307]
                        shift-right: [w310] -> w187
                        shift-left: w182 -> [w311]
                        tunnel: w170 -> [w304]
                        i -> [w308]
                        n81 = Add(x=w307, y=w308) -> (x+y=w305:i32)
                        n82 = Add(x=w304, y=w305) -> (x+y=w306:dbl)
                        n83 = Replace Array Subset(array=w311, new element=w309, index=w306) -> (w310:dbl[])
                      }
                      n84 = for {
                        N: w175 -> [_]
                        tunnel: w171 -> [w301]
                        shift-right: [w302] -> w176
                        shift-left: w180 -> [w303]
                        tunnel: w186 -> [w299]
                        tunnel: w170 -> [w296]
                        i -> [w300]
                        n85 = Add(x=w299, y=w300) -> (x+y=w297:i32)
                        n86 = Add(x=w296, y=w297) -> (x+y=w298:dbl)
                        n87 = Replace Array Subset(array=w303, new element=w301, index=w298) -> (w302:dbl[])
                      }
                      n88 = Add(x=w175, y=w186) -> (x+y=w172:i32)
                      n89 = local read "Y size"() -> (w159:i32)
                      n90 = for {
                        N: w174 -> [_]
                        shift-right: [w278] -> w185
                        shift-left: w187 -> [w279]
                        tunnel: w168 -> [w266]
                        tunnel: w172 -> [w272]
                        tunnel: w170 -> [w269]
                        i -> [w273]
                        n91 = local read "slope"() -> (w275:i16)
                        n92 = Add(x=w272, y=w273) -> (x+y=w271:i32)
                        n93 = Add(x=1, y=w273) -> (x+y=w276:i32)
                        n94 = Divide(x=w266, y=w275) -> (x/y=w274:dbl)
                        n95 = Add(x=w269, y=w271) -> (x+y=w270:dbl)
                        n96 = Multiply(x=w274, y=w276) -> (x*y=w267:dbl)
                        n97 = Subtract(x=w266, y=w267) -> (x-y=w268:dbl)
                        n98 = Replace Array Subset(array=w279, new element=w268, index=w270) -> (w278:dbl[])
                      }
                      n99 = Subtract(x=w159, y=1) -> (x-y=w158:i32)
                      n100 = Less?(x=w177, y=w158) -> (x < y?=w163:bool)
                      n101 = Add(x=w174, y=w172) -> (x+y=w169:i32)
                      n102 = case shown="假" w163 {
                        tunnel: [w194 w230] -> w161
                        tunnel: w176 -> [w201 w232]
                        tunnel: w174 -> [w202 w234]
                        tunnel: w173 -> [w197 w233]
                        tunnel: w170 -> [w198 w229]
                        tunnel: w172 -> [w199 w228]
                        tunnel: w171 -> [w200 w225]
                        tunnel: w170 -> [w196 w227]
                        tunnel: w169 -> [w195 w226]
                        frame False {
                          n103 = for {
                            N: w202 -> [_]
                            shift-right: [w223] -> w203
                            shift-left: w201 -> [w224]
                            tunnel: w198 -> [w222]
                            tunnel: w199 -> [w221]
                            tunnel: w200 -> [w212]
                            i -> [w218]
                            n104 = Add(x=w221, y=w218) -> (x+y=w220:i32)
                            n105 = Increment(x=w218) -> (x+1=w216:i32)
                            n106 = local read "slope"() -> (w215:i16)
                            n107 = Add(x=w222, y=w220) -> (x+y=w219:dbl)
                            n108 = Divide(x=w212, y=w215) -> (x/y=w217:dbl)
                            n109 = Multiply(x=w217, y=w216) -> (x*y=w214:dbl)
                            n110 = Subtract(x=w212, y=w214) -> (x-y=w213:dbl)
                            n111 = Replace Array Subset(array=w224, new element=w213, index=w219) -> (w223:dbl[])
                          }
                          n112 = for {
                            N: w197 -> [_]
                            shift-right: [w210] -> w194
                            shift-left: w203 -> [w211]
                            tunnel: w196 -> [w208]
                            tunnel: w195 -> [w206]
                            i -> [w209]
                            n113 = Add(x=w206, y=w209) -> (x+y=w207:i32)
                            n114 = Add(x=w208, y=w207) -> (x+y=w205:dbl)
                            n115 = Replace Array Subset(array=w211, new element=0, index=w205) -> (w210:dbl[])
                          }
                        }
                        frame True {
                          n116 = for {
                            N: w234 -> [_]
                            shift-right: [w256] -> w231
                            shift-left: w232 -> [w257]
                            tunnel: w229 -> [w255]
                            tunnel: w228 -> [w254]
                            tunnel: w225 -> [w246]
                            i -> [w251]
                            n117 = Add(x=w254, y=w251) -> (x+y=w253:i32)
                            n118 = local read "slope"() -> (w244:i16)
                            n119 = Increment(x=w251) -> (x+1=w248:i32)
                            n120 = Add(x=w255, y=w253) -> (x+y=w252:dbl)
                            n121 = Divide(x=1, y=w244) -> (x/y=w249:dbl)
                            n122 = Multiply(x=w249, y=w248) -> (x*y=w247:dbl)
                            n123 = Add(x=w246, y=w247) -> (x+y=w245:dbl)
                            n124 = Replace Array Subset(array=w257, new element=w245, index=w252) -> (w256:dbl[])
                          }
                          n125 = for {
                            N: w233 -> [_]
                            shift-right: [w242] -> w230
                            shift-left: w231 -> [w243]
                            tunnel: w227 -> [w240]
                            tunnel: w226 -> [w238]
                            tunnel: w225 -> [w235]
                            i -> [w241]
                            n126 = Increment(x=w235) -> (x+1=w236:i32)
                            n127 = Add(x=w238, y=w241) -> (x+y=w239:i32)
                            n128 = Add(x=w240, y=w239) -> (x+y=w237:dbl)
                            n129 = Replace Array Subset(array=w243, new element=w236, index=w237) -> (w242:dbl[])
                          }
                        }
                      }
                      n130 = for {
                        N: w173 -> [_]
                        shift-right: [w264] -> w162
                        shift-left: w185 -> [w265]
                        tunnel: w169 -> [w262]
                        tunnel: w170 -> [w259]
                        i -> [w263]
                        n131 = Add(x=w262, y=w263) -> (x+y=w261:i32)
                        n132 = Add(x=w259, y=w261) -> (x+y=w260:dbl)
                        n133 = Replace Array Subset(array=w265, new element=0, index=w260) -> (w264:dbl[])
                      }
                    }
                    frame True {
                      n134 = local read "Samples per spot"() -> (w317:i32)
                      n135 = Greater?(x=w314, y=0) -> (0:w312:bool)
                      n136 = case shown="真" w312 {
                        tunnel: [w338 w340] -> w316
                        tunnel: w315 -> [w338 w341]
                        frame False {
                        }
                        frame True {
                          n137 = Add(x="first", y=w341) -> (x+y=w340:dbl)
                        }
                      }
                      n138 = Subtract(x=w317, y=0) -> (x-y=w331:i32)
                      n139 = Subtract(x=w317, y="slope") -> (x-y=w324:i32)
                      n140 = Multiply(x=w317, y=w333) -> (x*y=w327:i32)
                      n141 = for {
                        N: w331 -> [_]
                        tunnel: w327 -> [w387]
                        shift-right: [w386] -> w329
                        shift-left: w332 -> [w385]
                        tunnel: w318 -> [w381]
                        i -> [w384]
                        n142 = Less?(x=w384, y=50) -> (x < y?=w382:bool)
                        n143 = case shown="真" w382 {
                          tunnel: w387 -> [_ w395]
                          tunnel: [w388 w394] -> w386
                          tunnel: w384 -> [_ w393]
                          tunnel: w385 -> [w388 w392]
                          tunnel: w381 -> [_ w389]
                          frame False {
                          }
                          frame True {
                            n144 = Add(x=w395, y=w393) -> (x+y=w390:i32)
                            n145 = Add(x=w389, y=w390) -> (x+y=w391:dbl)
                            n146 = Replace Array Subset(array=w392, new element=1.0 ("新元素/子数组"), index=w391) -> (w394:dbl[])
                          }
                        }
                      }
                      n147 = Subtract(x=w324, y="dwell time") -> (x-y=w323:i32)
                      n148 = for {
                        N: w317 -> [_]
                        tunnel: w334 -> [w402]
                        shift-right: [w403] -> w335
                        shift-left: w336 -> [w404]
                        tunnel: w327 -> [w400]
                        tunnel: w318 -> [w397]
                        i -> [w401]
                        n149 = Add(x=w400, y=w401) -> (x+y=w398:i32)
                        n150 = Add(x=w397, y=w398) -> (x+y=w399:dbl)
                        n151 = Replace Array Subset(array=w404, new element=w402, index=w399) -> (w403:dbl[])
                      }
                      n152 = for {
                        N: w323 -> [_]
                        tunnel: w316 -> [w410]
                        tunnel: w327 -> [w408]
                        shift-right: [w411] -> w328
                        shift-left: w337 -> [w412]
                        tunnel: w318 -> [w405]
                        i -> [w409]
                        n153 = Add(x=w408, y=w409) -> (x+y=w406:i32)
                        n154 = Add(x=w405, y=w406) -> (x+y=w407:dbl)
                        n155 = Replace Array Subset(array=w412, new element=w410, index=w407) -> (w411:dbl[])
                      }
                      n156 = Add(x=w323, y=w327) -> (x+y=w319:i32)
                      n157 = for {
                        N: "slope" -> [_]
                        shift-right: [w375] -> w326
                        shift-left: w328 -> [w376]
                        tunnel: w316 -> [w369]
                        tunnel: w319 -> [w368]
                        tunnel: w318 -> [w365]
                        tunnel: w314 -> [w359]
                        i -> [w362]
                        n158 = local read "slope"() -> (w371:i16)
                        n159 = Add(x=w368, y=w362) -> (x+y=w367:i32)
                        n160 = Equal?(x=w359, y=0) -> (x = y?=w361:bool)
                        n161 = Add(x=1, y=w362) -> (x+y=w373:i32)
                        n162 = Add(x=w365, y=w367) -> (x+y=w366:dbl)
                        n163 = case shown="真" w361 {
                          tunnel: [1 w378] -> w363
                          frame False {
                          }
                          frame True {
                            n164 = local read "first"() -> (w380:dbl)
                            n165 = Add(x=1, y=w380) -> (x+y=w378:dbl)
                          }
                        }
                        n166 = Divide(x=w363, y=w371) -> (x/y=w370:dbl)
                        n167 = Multiply(x=w370, y=w373) -> (x*y=w364:dbl)
                        n168 = Add(x=w369, y=w364) -> (x+y=w372:dbl)
                        n169 = Replace Array Subset(array=w376, new element=w372, index=w366) -> (w375:dbl[])
                      }
                      n170 = Add(x="slope", y=w319) -> (x+y=w321:i32)
                      n171 = for {
                        N: "dwell time" -> [_]
                        shift-right: [w353] -> w325
                        shift-left: w326 -> [w354]
                        tunnel: w321 -> [w351]
                        tunnel: w316 -> [w350]
                        tunnel: w318 -> [w346]
                        tunnel: w314 -> [w344]
                        i -> [w352]
                        n172 = Equal?(x=w344, y=0) -> (x = y?=w343:bool)
                        n173 = case shown="真" w343 {
                          tunnel: [1 w356] -> w342
                          frame False {
                          }
                          frame True {
                            n174 = local read "first"() -> (w358:dbl)
                            n175 = Add(x=1, y=w358) -> (x+y=w356:dbl)
                          }
                        }
                        n176 = Add(x=w350, y=w342) -> (x+y=w349:dbl)
                        n177 = Add(x=w351, y=w352) -> (x+y=w348:i32)
                        n178 = Add(x=w346, y=w348) -> (x+y=w347:dbl)
                        n179 = Replace Array Subset(array=w354, new element=w349, index=w347) -> (w353:dbl[])
                      }
                    }
                  }
                }
              }
            }
          }
          n180 = for {
            N: w55 -> [_]
            shift-right: [w70] -> w56
            shift-left: w57 -> [w71]
            tunnel: w54 -> [w69]
            tunnel: w51 -> [w66]
            i -> [w68]
            n181 = Add(x=w66, y=w68) -> (x+y=w67:dbl)
            n182 = Replace Array Subset(array=w71, new element=w69, index=w67) -> (w70:i32[])
          }
        }
      }
      "X index Array" <- w14
      "Y index Array" <- w13
      "Trigger" <- w12
      "nanoZ" <- w15
      "DO" <- w5
    }
    frame #1 {
      n183 = local read "Trigger"() -> (w458:dbl[])
      n184 = local read "Y index Array"() -> (w464:dbl[])
      n185 = local read "X index Array"() -> (w465:dbl[])
      n186 = local read "scan range (um)"() -> (w457:dbl)
      n187 = local read "first"() -> (w446:dbl)
      n188 = Multiply(x=w458, y="AmplitudeC") -> (x*y=w438:dbl[])
      "Trigger output" <- w438
      n189 = local read "nanoZ"() -> (w455:dbl[])
      n190 = Divide(x=w457, y=2) -> (x/y=w454:dbl)
      n191 = Multiply(x=w454, y=0.025) -> (x*y=w452:dbl)
      n192 = Subtract(x=w455, y=w452) -> (x-y=w442:dbl[])
      n193 = local read "X Size"() -> (w443:i32)
      n194 = Multiply(x="calibration", y=0.025) -> (x*y=w439:dbl)
      n195 = Subtract(x=w442, y=w439) -> (x-y=w421:dbl[])
      n196 = Add(x=w421, y=5) -> (x+y=w419:dbl[])
      "nanoZ output" <- w419
      n197 = Decrement(x=w443) -> (x-1=w444:i32)
      n198 = Divide(x="AmplitudeX", y=w444) -> (x/y=w450:dbl)
      n199 = Add(x=w444, y=w446) -> (x+y=w449:dbl)
      n200 = Multiply(x=w450, y=w449) -> (x*y=w447:dbl)
      n201 = local read "Y size"() -> (w436:i32)
      n202 = Add(x=w444, y=w446) -> (x+y=w445:dbl)
      n203 = Decrement(x=w436) -> (x-1=w472:i32)
      n204 = Divide(x=w465, y=w445) -> (x/y=w476:dbl[])
      n205 = Divide(x=w464, y=w472) -> (x/y=w467:dbl[])
      n206 = Subtract(x=w476, y=0.5) -> (x-y=w474:dbl[])
      n207 = Subtract(x=w467, y=0.5) -> (x-y=w469:dbl[])
      n208 = Multiply(x=w474, y=2) -> (x*y=w473:dbl[])
      n209 = Multiply(x=w469, y="AmplitudeY") -> (x*y=w470:dbl[])
      n210 = Multiply(x=w473, y=w447) -> (x*y=w463:dbl[])
      n211 = Multiply(x=w470, y=2) -> (x*y=w461:dbl[])
      n212 = Subtract(x=w463, y="zero point") -> (x-y=w432:dbl[])
      n213 = Subtract(x=w461, y="zero point 2") -> (x-y=w423:dbl[])
      n214 = call <vilib>:"Smoothing Filter Coefficients.vi"("fs"=100, "time constant"=1, "half-width"=20) -> ("forward coefficients"=w429:dbl[], "reverse coefficients"=w430:dbl[])  [unwired: 6 in, 1 out]
      n215 = call <vilib>:"Smoothing Filter Coefficients.vi"("fs"=100, "time constant"=1, "half-width"=20) -> ("forward coefficients"=w424:dbl[], "reverse coefficients"=w425:dbl[])  [unwired: 6 in, 1 out]
      n216 = call-poly <vilib>:"Zero Phase Filter.vi"("Forward Coefficients"=w429, "Reverse Coefficients"=w430, "X"=w432) -> ("Filtered X"=w431:dbl[])  [unwired: 7 in, 1 out]
      "X output Array" <- w431
      n217 = call-poly <vilib>:"Zero Phase Filter.vi"("Forward Coefficients"=w424, "Reverse Coefficients"=w425, "X"=w423) -> ("Filtered X"=w422:dbl[])  [unwired: 7 in, 1 out]
      "Y output Array" <- w422
      n218 = Build Array "Array creation"(w431, w422, w438, w419) -> (→"AO Data":dbl[][])
    }
    frame #2 {
      n219 = local read "Trigger output"() -> (w483:dbl[])
      n220 = local read "Trigger output"() -> (w485:dbl[])
      n221 = local read "nanoZ output"() -> (w478:dbl[])
      n222 = call <vilib>:"GetDateTimeInSecsCompatVI.vi"() -> ("double precision float"=w486:dbl)  [unwired: 1 in]
      "time" <- w486
      n223 = To Time Stamp(1:w486) -> (0:w479:timestamp)
      n224 = Bundle By Name("t0"=w479, "dt"="dt", "Y"=w485) -> (w482:waveform(dbl))  [unwired: 1 in]
      n225 = Bundle By Name("t0"=w479, "dt"="dt", "Y"=w483) -> (w481:waveform(dbl))  [unwired: 1 in]
      n226 = Bundle By Name("t0"=w479, "dt"="dt", "Y"=w478) -> (w477:waveform(dbl))  [unwired: 1 in]
      n227 = Build Array(w482, w481, w477) -> (→"Output Graph" →"XY Scan":waveform(dbl)[])
    }
  }
